vi "InitializeDlg.vi"(8 "error in (no error)":errorcluster, 10 "modes of operations":i8(ring)=1 items=["Profile Position Mode"=1, "Profile Velocity Mode"=3, "Homing Mode"=6, "Interpolated Position Mode"=7, "Position Mode"=-1, "Velocity Mode"=-2, "Current Mode"=-3, "Master Encoder Mode"=-5, "Step Direction Mode"=-6], 11 "nodeId":u16) -> (0 "error out":errorcluster, 3 "axis out":cluster{"keyHandle":u32, "nodeId":u16}={"keyHandle"=0, "nodeId"=1})   [LabVIEW 2018]
doc: "<B>InitializeDlg</B> registers available interfaces (CAN, USB and RS232) with which the EPOS can be operated and opens the selected interface for communication.\nThe function sets a new operational mode and clears all errors from a connected node."
panel:
  # "(c) 2007 - 2017 maxon motor ag.  ALL RIGHTS RESERVED."
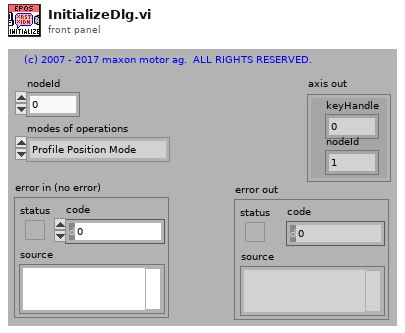
[diagram p1: front panel]
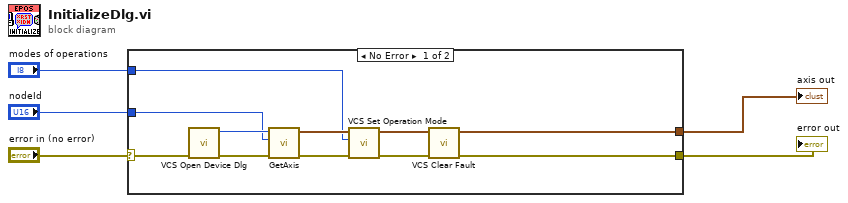
[diagram p0: block diagram]
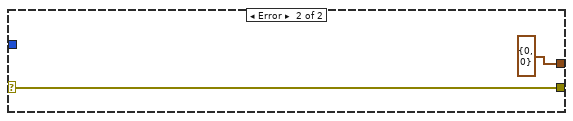
[diagram p2: hidden frame]
diagram:
  n1 = case shown="No Error" "error in (no error)" {
    selector: "error in (no error)" -> [w16 w18]
    tunnel: [w12 w18] -> w4
    tunnel: [w11 cluster{"keyHandle":u32, "nodeId":u16} {"keyHandle"=0, "nodeId"=0} ("axis out")] -> w3
    tunnel: "nodeId" -> [w7 _]
    tunnel: "modes of operations" -> [w6 _]
    frame No Error {
      n2 = call "VCS Open Device Dlg.vi"("error in (no error)"=w16) -> ("error out"=w15:errorcluster, "keyHandle out"=w8:u32)  [unwired: 9 in]
      n3 = call "GetAxis.vi"("error in (no error)"=w15, "nodeId"=w7, "keyHandle in"=w8) -> ("error out"=w14:errorcluster, "axis out"=w9:cluster{"keyHandle":u32, "nodeId":u16})  [unwired: 7 in]
      n4 = call "VCS Set Operation Mode.vi"("error in (no error)"=w14, "modes of operations"=w6, "axis in"=w9) -> ("error out"=w13:errorcluster, "axis out"=w10:cluster{"keyHandle":u32, "nodeId":u16})  [unwired: 7 in]
      n5 = call "VCS Clear Fault.vi"("error in (no error)"=w13, "axis in"=w10) -> ("error out"=w12:errorcluster, "axis out"=w11:cluster{"keyHandle":u32, "nodeId":u16})  [unwired: 8 in]
    }
    frame Error {
    }
  }
  "error out" <- w4
  "axis out" <- w3
